vi "Translator.Translate.Text.Buffer.FGV.vi"(6 "group":string, 7 "action":T1, 8 "error in":errorcluster, 9 "translated":string, 10 "text":string) -> (0 "error out":errorcluster, 1 "translated":string, 2 "found?":bool, 4 "ready":bool)   [LabVIEW 2019, in "Tools.lvlib"]
doc: "Stores the HW config data in memory. Let read it from memory (quick) instead of reading from file (slow) each time it is necessary."
uses:
  Tools.lvlib
  Translator.Translate.Text.Buffer.FGV.Action.ctl
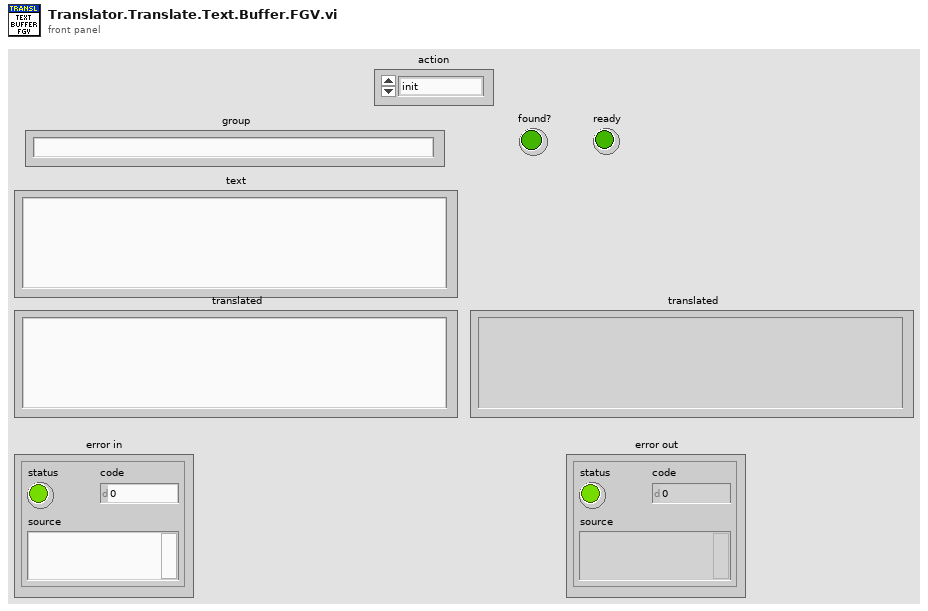
[diagram p1: front panel]
types:
  T1 = typedef "Tools.lvlib/Translator.Translate.Text.Buffer.FGV.Action.ctl" = enum16{"init", "get", "set"}
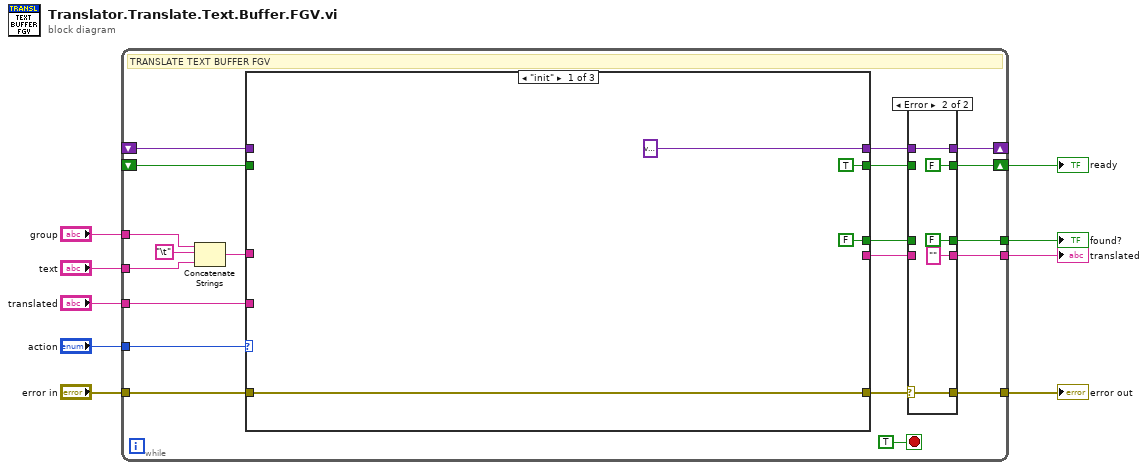
[diagram p0: block diagram]
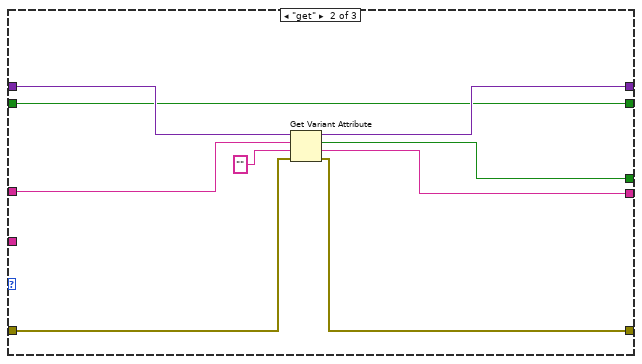
[diagram p3: hidden frame]
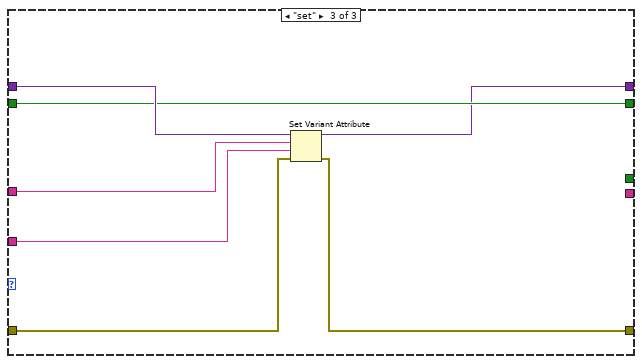
[diagram p4: hidden frame]
diagram:
  n1 = while {
    shift-right: [w19] -> _
    shift-left: _ -> [w28]
    tunnel: "error in" -> [w27]
    tunnel: [w10] -> w7
    shift-right: [w17] -> w9
    shift-left: _ -> [w26]
    tunnel: "action" -> [w25]
    tunnel: [w13] -> w1
    tunnel: [w15] -> w5
    tunnel: "translated" -> [w24]
    tunnel: "group" -> [w22]
    tunnel: "text" -> [w21]
    stop <- TRUE stop-if-true
    # "TRANSLATE TEXT BUFFER FGV"
    n2 = Concatenate Strings(w22, "\t", w21) -> (w20:string)
    n3 = case shown="\"init\"" w25 {
      tunnel: [variant w45 w54] -> w18
      tunnel: w28 -> [_ w52 w59]
      tunnel: [TRUE w44 w55] -> w16
      tunnel: w27 -> [w40 w49 w57]
      tunnel: [w40 w46 w56] -> w11
      tunnel: w26 -> [_ w44 w55]
      tunnel: w20 -> [_ w51 w58]
      tunnel: [_ w47 _] -> w12
      tunnel: [FALSE w48 _] -> w14
      tunnel: w24 -> [_ _ w53]
      frame "init" {
      }
      frame "get" {
        n4 = Get Variant Attribute(Variant=w52, name=w51, default value (empty Variant)="", error in=w49) -> (duplicate Variant=w45:variant, found=w48:bool, value=w47:string, error out=w46:errorcluster)
      }
      frame "set" {
        n5 = Set Variant Attribute(Variant=w59, name=w58, value=w53, error in=w57) -> (Variant out=w54:variant, error out=w56:errorcluster)  [unwired: 1 out]
      }
    }
    n6 = case shown="Error" w11 {
      selector: w11 -> [w30 w39]
      tunnel: [w34 w37] -> w19
      tunnel: w18 -> [w34 w37]
      tunnel: [w33 FALSE] -> w17
      tunnel: w16 -> [w33 _]
      tunnel: [w32 FALSE] -> w15
      tunnel: w14 -> [w32 _]
      tunnel: [w31 "" ("translated")] -> w13
      tunnel: w12 -> [w31 _]
      tunnel: [w30 w39] -> w10
      frame No Error {
      }
      frame Error {
      }
    }
  }
  "ready" <- w9
  "error out" <- w7
  "found?" <- w5
  "translated" <- w1
